vi "ConvertString_RollPitchYaw (SubVI).vi"(8 "error in (no error)":errorcluster, 11 "IMU String Data":string) -> (0 "error out":errorcluster, 3 "IMU Data Cluster":T1)   [LabVIEW 2016]
doc: "This VI accepts the string output from the RS232 port and outputs a cluster which contains Roll, Pitch, and Yaw data from the external IMU. An example of the expected string format is \"!ANG:-0.02,0.06,-0.04\"."
uses:
  Project Custom Controls/IMU Data Cluster.ctl
  <vilib>/regexp/Match Regular Expression.xnode
panel:
  # "Input Data"
  # "Output Data"
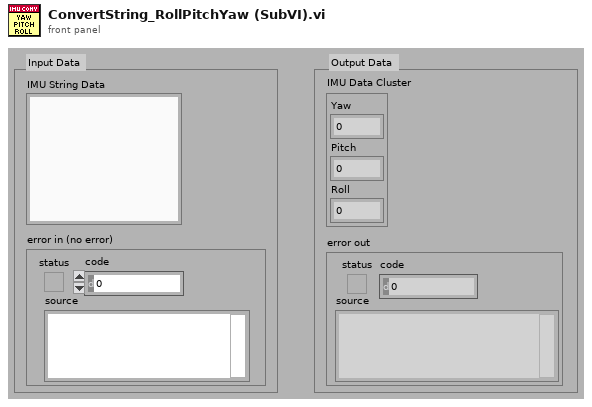
[diagram p1: front panel]
types:
  T1 = typedef "IMU Data Cluster.ctl" = cluster{"Yaw":dbl, "Pitch":dbl, "Roll":dbl}
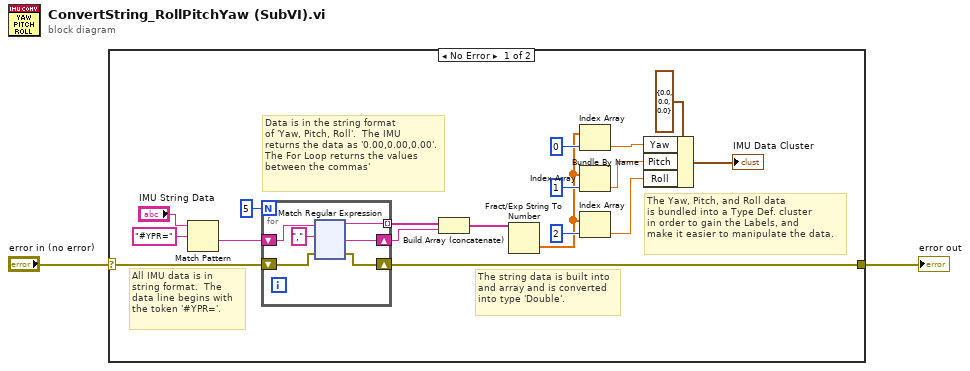
[diagram p0: block diagram]
diagram:
  n1 = case shown="No Error" "error in (no error)" {
    selector: "error in (no error)" -> [w6 w141]
    tunnel: [w14 w141] -> w2
    frame No Error {
      # "The Yaw, Pitch, and Roll data\nis bundled into a Type Def. cluster\nin order to gain the Labels, and\nmake it easier to manipulate the data."
      # "The string data is built into\nand array and is converted\ninto type 'Double'."
      # "Data is in the string format\nof 'Yaw, Pitch, Roll'.  The IMU\nreturns the data as '0.00,0.00,0.00'.\nThe For Loop returns the values\nbetween the commas'"
      # "All IMU data is in\nstring format.  The\ndata line begins with \nthe token '#YPR='."
      n2 = Match Pattern(string="IMU String Data", regular expression="#YPR=" ("search string/char (-)")) -> (after substring=w17:string)  [unwired: 1 in, 3 out]
      n3 = for {
        N: 5 -> [_]
        shift-right: [w24] -> w19
        shift-left: w17 -> [w26]
        tunnel: [w23] -> w18 mode=indexing
        shift-right: [w21] -> w14
        shift-left: w6 -> [w22]
        n4 = xnode "Match Regular Expression"("input string"=w26, "regular expression"=",", "error in"=w22) -> ("before match"=w23:string, "after match"=w24:string, "error out"=w21:errorcluster)  [unwired: 3 in, 2 out]
      }
      n5 = Build Array (concatenate)(w18, w19) -> (w20:string[])
      n6 = Fract/Exp String To Number(string=w20) -> (number=w10:dbl[])  [unwired: 3 in, 1 out]
      n7 = Index Array(array=w10, index=0) -> (element=w9:dbl)
      n8 = Index Array(array=w10, index=1) -> (element=w8:dbl)
      n9 = Index Array(array=w10, index=2) -> (element=w7:dbl)
      n10 = Bundle By Name(cluster=T1 {"Yaw"=0.0, "Pitch"=0.0, "Roll"=0.0} ("IMU Data"), "Yaw"=w9, "Pitch"=w8, "Roll"=w7) -> (→"IMU Data Cluster":T1)
    }
    frame Error {
      # "Skip all code if an error is detected\noutside this SubVI."
    }
  }
  "error out" <- w2
